vi "ArduinoLT-TimeAndTempature.vi"(8 "error in (no error)":errorcluster, 11 "Temperature":dbl) -> (0 "error out":errorcluster, 2 "double( Time, Temp )":dbl[](array[numeric]), 3 "str( Time, Temp )":string[](array[string]))   [LabVIEW 2016]
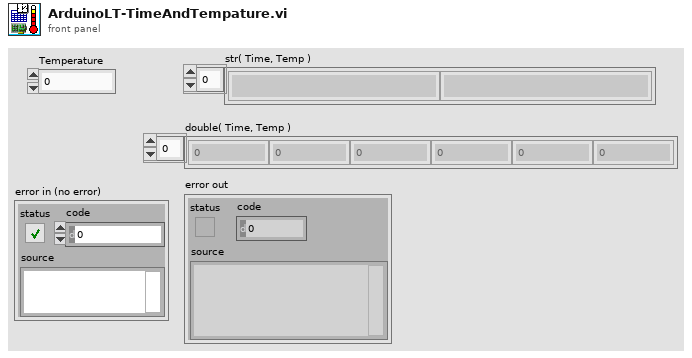
[diagram p1: front panel]
types:
  T1 = typedef "LVDateTimeRec.ctl" = cluster{"fractional second":dbl, "second":i32, "minute":i32, "hour":i32, "day of month":i32, "month":i32, "year":i32, "day of week":i32, "day of year":i32, "DST":i32}
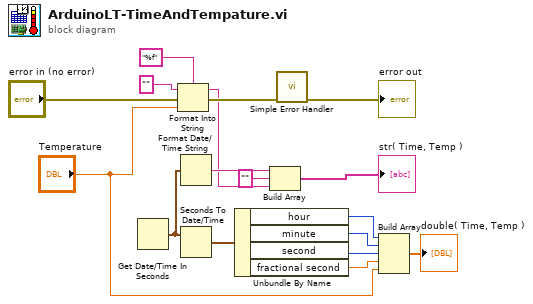
[diagram p0: block diagram]
diagram:
  n1 = Get Date/Time In Seconds() -> (seconds since 1Jan1904=w9:timestamp)
  n2 = Format Into String(format string="%f", initial string="", error in="error in (no error)", "Temperature") -> (resulting string=w2:string, error out=w4:errorcluster)
  n3 = Format Date/Time String(seconds (now)=w9) -> (date/time string=w11:string)  [unwired: 2 in]
  n4 = Seconds To Date/Time(time stamp (now)=w9) -> (date time rec=w10:T1)  [unwired: 1 in]
  n5 = Unbundle By Name(w10) -> ("hour"=w13:i32, "minute"=w14:i32, "second"=w15:i32, "fractional second"=w16:dbl)
  n6 = Build Array(w11, "" ("element"), w2) -> (→"str( Time, Temp )":string[])
  n7 = call <vilib>:"Simple Error Handler.vi"("error in (no error)"=w4) -> ("error out"=→"error out":errorcluster)  [unwired: 4 in, 4 out]
  n8 = Build Array(w13, w14, w15, w16, "Temperature") -> (→"double( Time, Temp )":dbl[])
